vi "Array Days Of The Week.vi"() -> ()   [LabVIEW 2012]
panel:
  out "The Day You Have Selected":string
  in  "Select A Day":dbl min=0.0 max=6.0 step=1.0
  out "Days Of The WeekArray":string[](array[string])
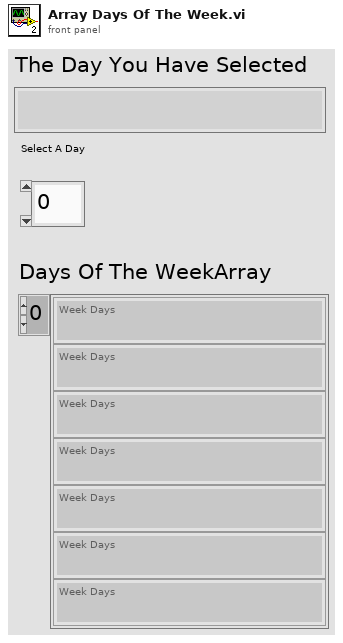
[diagram p1: front panel]
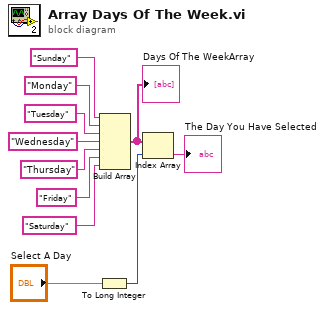
[diagram p0: block diagram]
diagram:
  n1 = To Long Integer(number="Select A Day") -> (32bit integer=w2:i32)
  n2 = Build Array("Sunday", "Monday", "Tuesday", "Wednesday", "Thursday", "Friday", "Saturday") -> (w3:string[])
  "Days Of The WeekArray" <- w3
  n3 = Index Array(array=w3, index=w2) -> (element=→"The Day You Have Selected":string)
